vi "ReciveParseMsg.vi"(8 "error in (no error)":errorcluster, 9 "timeout ms (25000)":i32, 11 "ServiceManager-Comms in":refnum<class "ServiceManager-Comms.lvclass">) -> (0 "error out":errorcluster, 2 "DownStreamMsgHandler":refnum<class "DownStreamMsgHandler.lvclass">, 3 "ServiceManager-Comms out":refnum<class "ServiceManager-Comms.lvclass">)   [LabVIEW 2020, in "ServiceManager.lvlib" / "ServiceManager-Comms.lvclass"]
uses:
  ServiceManager-Comms.lvclass
  ServiceManager/DownstreamMsg/DownStreamMsgHandler.lvclass
  ServiceManager-Comms.lvclass/ServiceManager-Comms.ctl
  2465c3ac-b30f-4f78-961d-aecd8e0bce88.vi
  <vilib>/JDP Science/JSONtext/String Subset.vi
  <vilib>/JDP Science/JSONtext/Parsing/Parse Full Path or Item Name.vi
  <vilib>/JDP Science/JSONtext/Next JSON Value.vi
  <vilib>/JDP Science/JSONtext/support/Error Cluster From Code.vi
  <vilib>/JDP Science/JSONtext/Offset/Find Item Locations by Path.vi
  <vilib>/JDP Science/JSONtext/JSON text to Variant.vi
  <vilib>/JDP Science/JSONtext/JSONtext.lvlib
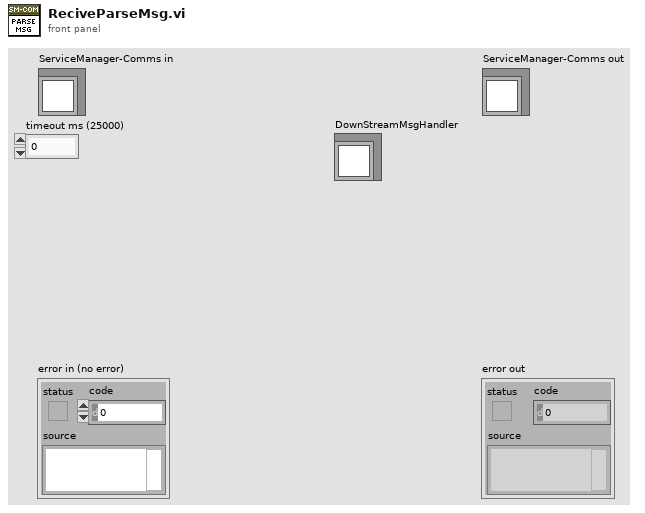
[diagram p1: front panel]
types:
  T1 = enum16{"Standard", "Buffered", "CRLF", "Immediate"}
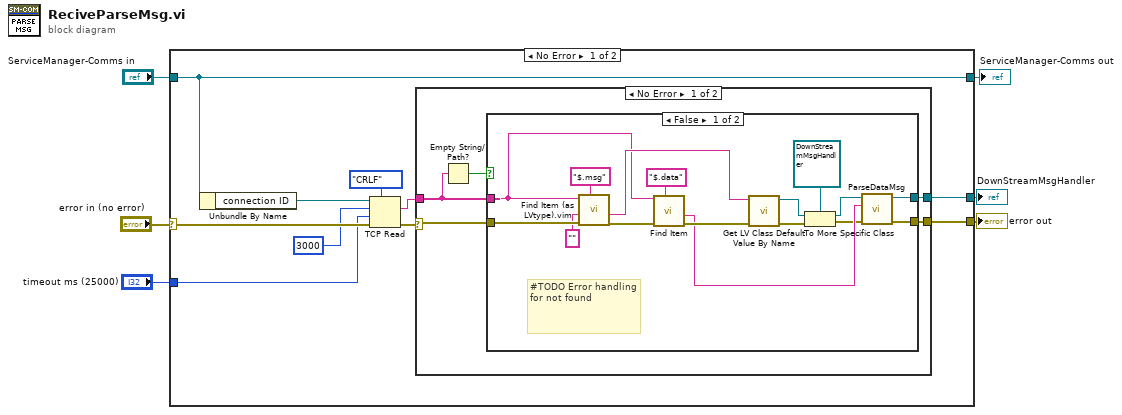
[diagram p0: block diagram]
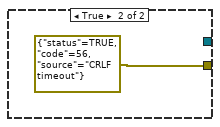
[diagram p2: hidden frame]
diagram:
  n1 = case shown="No Error" "error in (no error)" {
    selector: "error in (no error)" -> [w14 w41]
    tunnel: [w11 w41] -> w5
    tunnel: [w16 w40] -> w3
    tunnel: "ServiceManager-Comms in" -> [w16 w40]
    tunnel: [w10 _] -> w2
    tunnel: "timeout ms (25000)" -> [w9 _]
    frame No Error {
      n2 = Unbundle By Name(w16) -> ("connection ID"=w15:refnum<k5>)
      n3 = TCP Read(connection ID=w15, bytes to read=3000, error in (no error)=w14, 7:T1."CRLF" ("mode (standard)"), 9:w9) -> (data out=w12:string, error out=w13:errorcluster)  [unwired: 1 out]
      n4 = case shown="No Error" w13 {
        selector: w13 -> [w21 w39]
        tunnel: w12 -> [w18 _]
        tunnel: [w20 w39] -> w11
        tunnel: [w19 _] -> w10
        frame No Error {
          n5 = Empty String/Path?(string/path=w18) -> (empty?=w17:bool)
          n6 = case shown="False" w17 {
            tunnel: w21 -> [w37 _]
            tunnel: [w25 errorcluster {"status"=TRUE, "code"=56, "source"="CRLF timeout"} ("error out")] -> w20
            tunnel: [w24 _] -> w19
            tunnel: w18 -> [w22 _]
            frame False {
              # "#TODO Error handling for not found"
              n7 = call "Find Item (as LVtype).vim"("$Path or Item Name"="$.msg", "error in (no error)"=w37, "Data Type and Default Value"="", "JSON"=w22) -> ("error out"=w30:errorcluster, "Data"=w23:string)  [unwired: 4 in, 2 out]
              n8 = call <vilib>:"Find Item.vi"("$Path or Item Name"="$.data", "error in (no error)"=w30, "JSON"=w22) -> ("error out"=w29:errorcluster, "<JSON>"=w27:string)  [unwired: 5 in, 2 out]
              n9 = call <vilib>:"Get LV Class Default Value By Name.vi"("error in (no error)"=w29, "class name"=w23) -> ("error out"=w34:errorcluster, "object"=w33:refnum<class>)  [unwired: 8 in]
              n10 = To More Specific Class(target class=refnum<class "DownStreamMsgHandler.lvclass"> refnum ("DownstreamMsg.lvlib:DownStreamMsgHandler.lvclass"), reference=w33, error in=w34) -> (specific class reference=w31:refnum<class "DownStreamMsgHandler.lvclass">, error out=w26:errorcluster)
              n11 = call-dynamic "ParseDataMsg.vi"("error in (no error)"=w26, "JSON<>"=w27, "DownStreamMsgHandler in"=w31) -> ("error out"=w25:errorcluster, "DownStreamMsgHandler out"=w24:refnum<class "DownStreamMsgHandler.lvclass">)  [unwired: 7 in]
            }
            frame True {
            }
          }
        }
        frame Error {
        }
      }
    }
    frame Error {
    }
  }
  "error out" <- w5
  "ServiceManager-Comms out" <- w3
  "DownStreamMsgHandler" <- w2
